vi "Gel Tugging Force Mode_Data Logger v16.20 EPI.vi"() -> ()   [LabVIEW 2015]
uses:
  <vilib>/Utility/error.llb/DialogType.ctl
  <vilib>/DAQmx/read.llb/DAQmx Read (Analog 2D DBL NChan NSamp).vi
  <vilib>/DAQmx/create/channels.llb/DAQmx Create Channel (AI-Voltage-Basic).vi
  <vilib>/DAQmx/configure/timing.llb/DAQmx Timing (Sample Clock).vi
  <vilib>/DAQmx/configure/trigger.llb/DAQmx Start Trigger (Digital Edge).vi
  <vilib>/DAQmx/miscellaneous.llb/DAQmx Fill In Error Info.vi
  <vilib>/Utility/file.llb/Write Delimited Spreadsheet (DBL).vi
  <resource>/objmgr/daqmx.rc
  <resource>/objmgr/ni.dex.rc
panel:
  in  "Filename: 2":string="R1"
  out "Loop Index":i32
  out "Data Points":u64
  in  "Working Directory":path=path "C:/Users/Selby1/Desktop" caption="Path"
  in  "Filename:":string="S20210722_1mgmL_37C-S2-B1-EDC"
  out "Current Plot (V)":dbl[](graph)
  out "Exposure Plot (V)":dbl[](graph)
  out "Flux Plot (V)":dbl[](graph)
  in  "Start Manual Trigger Button":bool
  in  "Trigger Type?":bool=TRUE
  in  "Notes:":string="0.5-µm carboxylate-coated Fluorosphere red beads\n4.5-µm M450 Dynabeads tosylactivated magnetic beads \n0.75 mg/mL type I collagen gel @ 37°C, pH ~7.4. Prepared on 2021-08-17\nNOT Covered with 2.6mM EDAC + 0.1M MES (pH~ 6.0) solution for 30 minutes\n18-mm diameter Sylgard 184 1:10 mixture. Poured 6.2 g onto \"100-mm\" petri dish to create ~750 µm thick molds.\nCoated the gel with 10 µL red bead/mL MilliQ water left for 10-30 seconds. \nWashed the gel before adding the red beads with clean milliQ water\n250 µL of collagen gel mix (~800 µm). Consider using 235 µL next time."
  out "Total Ramp \nTime (ms)":i16
  out "# Ramp\nSteps":i16
  out "Red Fluoroescent Microspheres\nDiameter (Micron)":dbl=0.5 format="%#.1g"
  out "Tip Initial XY Separation\n (micron) Separation\n Distance (micron)":dbl=15.0
  out "Image Scale \n(micron/pixel)":dbl=0.21604
  out "Gel Thickness\n(Micron)":dbl=662.0
  in  "Fluoro Beads \nZ-Level\n(Micron)":dbl
  in  "Magnetic \nBead Z-Level\n(Micron)":dbl
  out "Tip Z-level Above Gel Surface (micron)":dbl=11.0
  out "Digital Trigger":bool
  out "Flux On\n Setpoint (Gs)":dbl=2.4945191 format="%.3g"
  out "Column 4":string="Flux Sensor (V)"
  out "Column 3":string="Flux Sensor (V)"
  out "Column 1":string="Flux Sensor (V)"
  out "Column 2":string="Flux Sensor (V)"
  out "Temperature\n(ºC)":dbl=25.7
  out "Ready?":bool
  in  "?":bool
  out "Relative \nHumidity (%)":dbl=42.0
  out "Magnetic Flux Sensor\n Sensitivity (V/Gs)":dbl=2.4945191 format="%#_8g"
  out "Magnetic Bead\nDiameter (Micron)":dbl=4.5 format="%#.1g"
  out "Needle\n Inclination \nAngle (º)":dbl=25.0
  out "Cycles":i16
  out "Downloading\nData":bool
  out "Magnetic Flux Sensor\n Zero, Crude Mean (V)":dbl=2.4945191 format="%.6g"
  # "For Gel Tugging Experiments v16.20-EPI Part"
  # "Verify Data Further with  \"Gel Tugging Force Mode_Data Reduction v16.00.vi\" or \"ReadSensorData.m\" in MATLAB"
  # "Step 1: Enter:"
  # "-EPI-"
  # ".dat"
  # "&"
  # "_Notes.txt"
  # "Manual"
  # "Automatic"
  # "Step 2: Click TRGR or Run Macro in Nikon Elements"
  # "datapoints downloaded"
  # "out of"
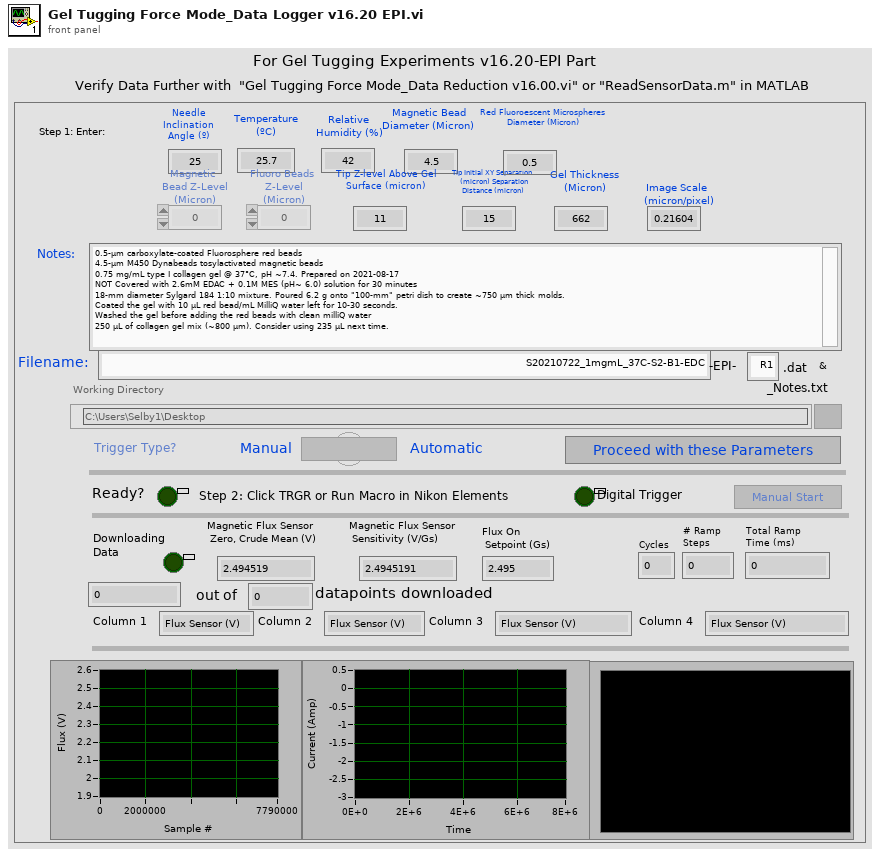
[diagram p1: front panel]
types:
  T1 = enum8{"Enabled", "Disabled", "Disabled and Grayed Out"}
  T2 = typedef "DialogType.ctl" = u16
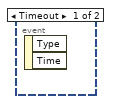
[diagram p2: hidden frame]
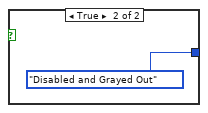
[diagram p3: hidden frame]
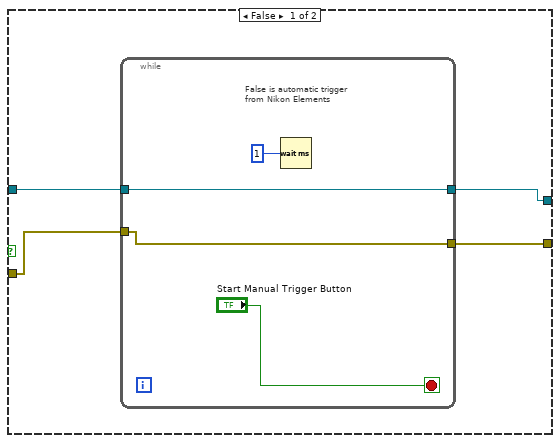
[diagram p4: hidden frame]
diagram:
  # "Modified from v15.00 by #Waddah #Moghram on 12/18/2018 and thereafter.\n1. Added a note section that will be in a file with the same note, but add \"notes\" to it. \n2. Tip -> Magnetic Bead. Magnetic Bead -> Fluorobeads. Fluoro beads -> Tip z-level. Headers were corrected 12/20/2018\n \nModified from v11.00 by #Waddah #Moghram on 5/4/2018 and thereafter:\n1. Updated the header to include gel-related information such as z-levels for the tip, bead, and thickness; gel thickness.\n2. Changed output file extension to *.dat\n3. Added a few other headers. Updated Ramp Step Information 11/28/2018\n\nModified from v10.00 by #Waddah #Moghram on 4/26/2018:\n1. This program will get the digital trigger from Nikon Elements. Then it will forward it to the control sequence VI on the slave DAQ for real-time sequence. This is a roundabout way to deal with the issue of ground loop problems.\n\nModified from v8.00 and later by #Waddah #Moghram on 4/4/2018 \n2. Just add an extra Row...with Null Flux Corrective just for the record. Did not mess with anything previously\n2. \"Flux Observed Zero\" renamed to \"Null Flux Observed\"\n3. \"AO Signal\" is replaced back to \"Camera Exposure (V)\"\n4. Added Labels \"Rows\" to the Header to keep track\n5. Updated Samples read per loop from 400 to 40000 4/1/2018\n6. Added Headers for Gel properties\n\nModified from v7.40 by #Waddah #Moghram on 1/4/2018\n1. Remove Step 0: Recording temperature with thermocouple. Thermocouple reading is not reliable, whether is the one built into labVIEW or the handheld one. Enter the value read by the Digital Thermometer along with relative humidity readings.\n2. Added an extra row to store both sets of PIDs for ON/OFF. \n3. Modified Tabbing Order on 3/4/2018\n4. Added Columns Display at front panel 3/18/2018\n\nModified from v7.30 by #Waddah #Moghram on 12/23/2017\n1. Added event close loop to make the Data Logger Running False if user closes it abruptly. \nNote: Aborting event is not included. Avoid aborting if possible.\n2. corrected total number of data points to allow for more than 2 seconds 1/4/2018 by #WIM\n\nModified from v7.00 by #Waddah #Moghram on 12/21/2017\n1. Reduce Thermocouple time to 1 \n2. Added another Text to record room temperature manual. But be consistent.\n\nModified from v6.00 by #Waddah #Moghram on 12/18/2017\n1. Added Relative Humidity Entry instead of \"Dummy Variable Entry in the Header.\" This value is to be entered from the reading of Relative Humidity\\\n2. Added Thermocouple measurement VI into this one. Average and storage into Data Logger for future purposes. \n\nModified from v5.22 by #Waddah #Moghram on 12/05/2017\n1. Added Entry for Magnetic Sensor Sensitivity\n2. Added Precisions for Header Values\n\nModified from v.4.00 by #Waddah #Moghram on 8/9/2017\n\nModified from v.3.80 by #Waddah #Moghram on 8/7/2017\n*Current Dialog boxes. Use Stacked sequences. Cleaned up v.3.80\n*Included Post  & Pre-wave Periods in Data Collection\n\nModified by #Waddah #Moghram on 8/7/2017\n*Include PID Parameters in the file\n*Modified headers of columns to be able to be extracted from MATLAB\n*Network stream loop is cleaned up \n*Removed Data Logging Time. Whatever it it takes to download the entire stream.\n*works with local single process FIFO\n\nDigital Input (Trigger)\n1. Dev3/PFI0 is connected internally in the DAQ-1/Master Connecter block. It is also wired up to DAQ-2/Slave Connector Block\n\nModifications from previous edition:\n1. Removed AI1 & AI2 to see if instability is due to a ground loop.\n\nNote: Sampling rate for Data Logger is 10,000 Samples/Second"
  n1 = flat-sequence {
    tunnel: [w20] -> w2
    tunnel: [w32] -> w12
    tunnel: [w33] -> w11
    tunnel: w2 -> [w29]
    tunnel: [w29] -> w1
    tunnel: w12 -> [w46]
    tunnel: w11 -> [w45]
    tunnel: [w47] -> w7
    tunnel: [w48] -> w3
    tunnel: w1 -> [w44]
    tunnel: [w228] -> w8
    tunnel: w7 -> [w161]
    tunnel: [w161] -> w6
    tunnel: [w291] -> w5
    tunnel: [w167] -> w4
    tunnel: w3 -> [w291]
    tunnel: w8 -> [w301]
    tunnel: w6 -> [w307]
    tunnel: [w296] -> w10
    tunnel: w5 -> [w306]
    tunnel: [w300] -> w9
    tunnel: w4 -> [w315]
    tunnel: w10 -> [w382]
    tunnel: w9 -> [w381]
    frame #0 {
      (unwired) "1. OPEN the PID Control VI & Follow Instructions **if you have not done so already**.\n2. Click OK to begin temperature measurement & ENTER other variables afterwards.\n3. RUN the macro (if a macro is used). Otherwise, CLICK  \"TRGR\" button in Nikon Elements to initiate Fast Timelapse Image Capture, Data Acquisition, and PID-Controlled Sequence."
      # "Clear Graphs"
      # "Reset the Data Download"
      n2 = shared-variable "NI-GenericDesktopPC-3A84958E\\Kopco PS Project Target Variables Library.lvlib\\DataFolderName"() -> (w14:string)  [unwired: 1 in, 1 out]
      n3 = shared-variable "NI-GenericDesktopPC-3A84958E\\Kopco PS Project Target Variables Library.lvlib\\DataFileName"() -> (w15:string)  [unwired: 1 in, 1 out]
      n4 = shared-variable "NI-GenericDesktopPC-3A84958E\\Kopco PS Project Target Variables Library.lvlib\\Notes"() -> (w19:string)  [unwired: 1 in, 1 out]
      n5 = String To Path(string=w14) -> (path=w13:path)
      n6 = property on="Exposure Plot (V)" class="WFGraph (strict)"("Value"=dbl[] [] ("Current Plot (V)")) -> ()  [unwired: 2 in, 2 out]
      n7 = property on="Current Plot (V)" class="WFGraph (strict)"("Value"=dbl[] [] ("Flux Plot (V)")) -> ()  [unwired: 2 in, 2 out]
      n8 = property on="Flux Plot (V)" class="WFGraph (strict)"("Value"=dbl[] [] ("Exposure Plot (V)")) -> ()  [unwired: 2 in, 2 out]
      n9 = property on="Notes:" class="Str"("Text.Text"=w19) -> ()  [unwired: 2 in, 2 out]
      n10 = property on="Filename:" class="Str"("Text.Text"=w15) -> ()  [unwired: 2 in, 2 out]
      n11 = property on="Working Directory" class="Path"("Value"=w13) -> ()  [unwired: 2 in, 2 out]
    }
    frame #1 {
      # "Gives a pause to adjust the values before confirmation"
      # "Bound to \"Experiment Settings Entered\"\nglobal shared variable."
      n12 = while {
        tunnel: ["?"] -> w21
        tunnel: ["Trigger Type?"] -> w20
        stop <- "?" stop-if-true
        w23 = FALSE ("Data Download")
        n13 = shared-variable "NI-GenericDesktopPC-3A84958E\\Kopco PS Project Target Variables Library.lvlib\\Data Download"(w23) -> ()  [unwired: 1 in, 1 out]
        n14 = shared-variable "NI-GenericDesktopPC-3A84958E\\Kopco PS Project Target Variables Library.lvlib\\Data Logger Running"(TRUE ("Data Logger Running")) -> ()  [unwired: 1 in, 1 out]
        n15 = case shown="False" "Trigger Type?" {
          tunnel: [T1."Enabled" ("Disabled") T1."Disabled and Grayed Out" ("Disabled")] -> w26
          frame False {
          }
          frame True {
          }
        }
        n16 = shared-variable "NI-GenericDesktopPC-3A84958E\\Kopco PS Project Target Variables Library.lvlib\\Temperature Measured"(w23) -> ()  [unwired: 1 in, 1 out]
        n17 = shared-variable "NI-GenericDesktopPC-3A84958E\\Kopco PS Project Target Variables Library.lvlib\\Experiment Settings Entered"(w23) -> ()  [unwired: 1 in, 1 out]
        n18 = shared-variable "NI-GenericDesktopPC-3A84958E\\Kopco PS Project Target Variables Library.lvlib\\Digital Trigger"(w23) -> ()  [unwired: 1 in, 1 out]
        n19 = property on="Start Manual Trigger Button" class="Bool"("Disabled"=w26) -> ()  [unwired: 2 in, 2 out]
      }
      n20 = shared-variable "NI-GenericDesktopPC-3A84958E\\Kopco PS Project Target Variables Library.lvlib\\Experiment Settings Entered"(w21) -> ()  [unwired: 1 in, 1 out]
    }
    frame #2 {
      w30 = 30000.0  # AI Frequency
      w34 = 10106 items=["Default"=-1, "RSE"=10083, "NRSE"=10078, "Differential"=10106, "Pseudodifferential"=12529] ("input terminal configuration")
      w35 = 10123 items=["Finite Samples"=10178, "Continuous Samples"=10123] ("sample mode")
      # "Configuring Analog Inputs (AIs)\n3. Dev2/AI5 is connected to \"RAW\" Magnetic Flux Sensor\n4. Dev2/AI6 is connected to \"Current Senssor (1A/V)\"\n5. Dev2/AI7 is connected to Camera Exposure Signal (\"Out 4\" on sCMOS Camera)"
      # "As of 8/3/2017. This is \njust to initiate digital trigger.\nNo data is collected via master DAQ"
      n21 = call-poly <vilib>:"DAQmx Create Virtual Channel.vi"("maximum value"=10.0, "minimum value"=-10.0, "input terminal configuration"=w34, "physical channels"="Dev3/ai3") -> ("task out"=w37:refnum<k21>, "error out"=w36:errorcluster)  [unwired: 10 in]
      n22 = call-poly <vilib>:"DAQmx Timing.vi"("task/channels in"=w37, "sample mode"=w35, "rate"=w30, "source"=tag "OnboardClock" ("Sample Clock Source"), "error in"=w36) -> ("task out"=w38:refnum<k21>, "error out"=w39:errorcluster)  [unwired: 9 in]
      n23 = call <vilib>:"DAQmx Configure Input Buffer.vi"("task/channels in"=w38, "buffer size (in samples per channel)"=200000, "error in"=w39) -> ("task out"=w32:refnum<k21>, "error out"=w33:errorcluster)  [unwired: 11 in]
    }
    frame #3 {
      n24 = case shown="True" w44 {
        tunnel: [w52 w70] -> w49
        tunnel: w45 -> [w53 w62]
        tunnel: [w55 w61] -> w50
        tunnel: w46 -> [w54 w60]
        frame False {
          n25 = while {
            tunnel: [w58] -> w55
            tunnel: w54 -> [w58]
            tunnel: w53 -> [w57]
            tunnel: [w57] -> w52
            stop <- "Start Manual Trigger Button" stop-if-true
            # "False is automatic trigger \nfrom Nikon Elements"
            n26 = Wait (ms)(milliseconds to wait=u32 1) -> ()  [unwired: 1 out]
          }
        }
        frame True {
          w63 = 10280 items=["Rising"=10280, "Falling"=10171] ("edge")
          # "True is automatic trigger \nfrom Nikon Elements"
          # "Waiting for Digital Trigger (\"TRGR\") from Nikon Element\nOr Macro that has a digital trigger"
          n27 = call-poly <vilib>:"DAQmx Trigger.vi"("task/channels in"=w60, "source"=tag "/Dev3/PFI0", "edge"=w63, "error in"=w62) -> ("task out"=w65:refnum<k21>, "error out"=w67:errorcluster)  [unwired: 10 in]
          n28 = property class="DAQmx Trigger"(reference=w65, error in=w67, "Start.DigEdge.DigFltr.MinPulseWidth"=1e-06) -> (reference out=w66:refnum<k21>, error out=w68:errorcluster)
          n29 = call <vilib>:"DAQmx Start Task.vi"("task/channels in"=w66, "error in"=w68) -> ("task out"=w61:refnum<k21>, "error out"=w70:errorcluster)  [unwired: 12 in]
        }
      }
      n30 = while "Just a one-item loop for to start the digital trigger" {
        tunnel: w49 -> [w77]
        tunnel: w50 -> [w76]
        tunnel: [w75] -> w48
        tunnel: [w74] -> w47
        tunnel: [w71] -> w51
        i -> [w73]
        stop <- w71 stop-if-true
        w79 = -1.0  # timeout
        # "Added on 4/24/2018. Digital Trigger to be transferred to \nRT control sequence VI"
        n31 = Equal?(x=1, y=w73) -> (x = y?=w71:bool)
        n32 = call-poly <vilib>:"DAQmx Read.vi"("task/channels in"=w76, "number of samples per channel"=1, "timeout"=w79, "error in"=w77) -> ("task out"=w75:refnum<k21>, "error out"=w74:errorcluster)  [unwired: 9 in, 1 out]
        n33 = Unbundle By Name(w74) -> ()  [unwired: 1 out]
      }
      n34 = shared-variable "NI-GenericDesktopPC-3A84958E\\Kopco PS Project Target Variables Library.lvlib\\Digital Trigger"(w51) -> ()  [unwired: 1 in, 1 out]
    }
    frame #4 {
      w117 = 0.0  # number
      w133 = "\t"
      w135 = "\t"
      w158 = "\t"
      w157 = "\t"
      w172 = "\t"
      w171 = "\t"
      (unwired) "AO Signal (V)" ("string")
      w192 = "\t"
      w190 = "\t"
      w218 = "\t"
      w216 = "\t"
      w277 = "\t"
      w275 = "\t"
      w243 = "\t"
      w241 = "\t"
      w178 = "Current AO (V)" ("string")
      w257 = "\t"
      w260 = "\t"
      w169 = "Camera Exposure TTL (V)" ("string")
      w254 = "\t"
      w177 = "Current Sensor (V or A)" ("string")
      w253 = "Flux Sensor (V)" ("string")
      # "Added on 3/17/2018\nfor mini DeGauss & \ntuning experiments. \nModify controller Program accordingly.\n4/4/2018. Back to Camera Exposure"
      # "Added on 3/17/2018\nfor mini DeGauss & \ntuning experiments. \nModify controller Program accordingly.\n4/4/2018. Back to Camera Exposure"
      # "Step Duration is changed to \nSampling Rate, 1/5/2018 by WIM"
      # "Sampling Rate (samples/sec)"
      # "Removed (%) on 12/20/2017 @ 6:58 PM.\nIt should not be % since it is alreayd in decimal. Otherwise, it is %"
      # "Changed from (mV/Gs) to (V/Gs) on 7/18/2017"
      # "Modified on 7/19/2017 to Including Sampling Frequency \ninstead of Sampling Rate to minimize round off Error"
      # "3rd Line Header"
      # "Magentic Sensor Sensitivity"
      n35 = shared-variable "NI-GenericDesktopPC-3A84958E\\Kopco PS Project Target Variables Library.lvlib\\Flux Setpoint ON Gs Relative"() -> (w164:dbl)  [unwired: 1 in, 1 out]
      "Flux On\n Setpoint (Gs)" <- w164
      n36 = shared-variable "NI-GenericDesktopPC-3A84958E\\Kopco PS Project Target Variables Library.lvlib\\NeedleInclinationAngle"() -> (w96:dbl)  [unwired: 1 in, 1 out]
      "Needle\n Inclination \nAngle (º)" <- w96
      n37 = shared-variable "NI-GenericDesktopPC-3A84958E\\Kopco PS Project Target Variables Library.lvlib\\MagneticBeadDiameterMicron"() -> (w95:dbl)  [unwired: 1 in, 1 out]
      "Magnetic Bead\nDiameter (Micron)" <- w95
      n38 = shared-variable "NI-GenericDesktopPC-3A84958E\\Kopco PS Project Target Variables Library.lvlib\\Temperature"() -> (w97:dbl)  [unwired: 1 in, 1 out]
      "Temperature\n(ºC)" <- w97
      n39 = shared-variable "NI-GenericDesktopPC-3A84958E\\Kopco PS Project Target Variables Library.lvlib\\Null Flux Pre Period"() -> (w288:dbl)  [unwired: 1 in, 1 out]
      n40 = shared-variable "NI-GenericDesktopPC-3A84958E\\Kopco PS Project Target Variables Library.lvlib\\RelativeHumidity"() -> (w94:dbl)  [unwired: 1 in, 1 out]
      "Relative \nHumidity (%)" <- w94
      n41 = shared-variable "NI-GenericDesktopPC-3A84958E\\Kopco PS Project Target Variables Library.lvlib\\Zero Flux Observed GS"() -> (w287:dbl)  [unwired: 1 in, 1 out]
      n42 = shared-variable "NI-GenericDesktopPC-3A84958E\\Kopco PS Project Target Variables Library.lvlib\\Null Flux Post Period"() -> (w289:dbl)  [unwired: 1 in, 1 out]
      n43 = shared-variable "NI-GenericDesktopPC-3A84958E\\Kopco PS Project Target Variables Library.lvlib\\PID Parameters ON"() -> (w230:dbl[])  [unwired: 1 in, 1 out]
      n44 = shared-variable "NI-GenericDesktopPC-3A84958E\\Kopco PS Project Target Variables Library.lvlib\\Sensor Sensitivity Core"() -> (w213:dbl)  [unwired: 1 in, 1 out]
      "Magnetic Flux Sensor\n Sensitivity (V/Gs)" <- w213
      n45 = shared-variable "NI-GenericDesktopPC-3A84958E\\Kopco PS Project Target Variables Library.lvlib\\Zero Flux Calibrated Core"() -> (w261:dbl)  [unwired: 1 in, 1 out]
      "Magnetic Flux Sensor\n Zero, Crude Mean (V)" <- w261
      n46 = Index Array(array=w230, index=3) -> (element=w290:dbl)
      n47 = Index Array(array=w230, index=4) -> (element=w167:dbl)
      n48 = Index Array(array=w230, index=2) -> (element=w234:dbl)
      n49 = Number To Fractional String "Flux ON Relative Setpoint (Gs)"(number=w164) -> (F-format string=w282:string)  [unwired: 3 in]
      n50 = Number To Fractional String "Flux Observed Zero (Gs)"(number=w287) -> (F-format string=w281:string)  [unwired: 3 in]
      n51 = Index Array(array=w230, index=1) -> (element=w237:dbl)
      n52 = Index Array(array=w230, index=0) -> (element=w239:dbl)
      n53 = Number To Fractional String "Pre- Zero Interval (s)"(number=w288) -> (F-format string=w280:string)  [unwired: 3 in]
      n54 = Number To Fractional String "Post- Zero Interval (s)"(number=w289) -> (F-format string=w276:string)  [unwired: 3 in]
      n55 = Divide(x=w94, y=100.0) -> (x/y=w207:dbl)
      n56 = shared-variable "NI-GenericDesktopPC-3A84958E\\Kopco PS Project Target Variables Library.lvlib\\Cycles"() -> (w273:i16)  [unwired: 1 in, 1 out]
      n57 = shared-variable "NI-GenericDesktopPC-3A84958E\\Kopco PS Project Target Variables Library.lvlib\\PID Parameters OFF"() -> (w176:dbl[])  [unwired: 1 in, 1 out]
      n58 = Number To Fractional String "Proportional Gain (K_c)"(number=w239) -> (F-format string=w249:string)  [unwired: 3 in]
      n59 = Number To Exponential String "Integral Time (T_i, min)"(number=w237) -> (E-format string=w248:string)  [unwired: 3 in]
      n60 = shared-variable "NI-GenericDesktopPC-3A84958E\\Kopco PS Project Target Variables Library.lvlib\\Needle Used"() -> (w179:i8)  [unwired: 1 in, 1 out]
      n61 = Number To Fractional String "Magnetic Sensor Mean, Crude"(number=w261, precision (6)=i16 6) -> (F-format string=w264:string)  [unwired: 2 in]
      n62 = Number To Exponential String "Derivative Time (T_d, min)"(number=w234) -> (E-format string=w247:string)  [unwired: 3 in]
      n63 = Number To Fractional String "Samples Pushed to PID at a time"(number=w290, precision (6)=i16 0) -> (F-format string=w242:string)  [unwired: 2 in]
      n64 = Number To Fractional String "Number of Cycles"(number=w273, precision (6)=i16 0 ("width (-)")) -> (F-format string=w262:string)  [unwired: 2 in]
      n65 = Number To Fractional String "Sampling Rate (Samples/Sec)"(number=w167, precision (6)=i16 0) -> (F-format string=w256:string)  [unwired: 2 in]
      n66 = Number To Fractional String "Mean Temperature (ºC)"(number=w97, precision (6)=i16 1) -> (F-format string=w223:string)  [unwired: 2 in]
      n67 = Number To Fractional String "Inclination Angle (º)"(number=w96, precision (6)=i16 0) -> (F-format string=w222:string)  [unwired: 2 in]
      n68 = Number To Fractional String "Relative Humidity (%)"(number=w207, precision (6)=i16 2 ("width (-)")) -> (F-format string=w217:string)  [unwired: 2 in]
      n69 = Number To Fractional String "Magnetic Bead Diameter (Micron)"(number=w95, precision (6)=i16 1) -> (F-format string=w221:string)  [unwired: 2 in]
      n70 = Number To Fractional String "Magnetic Sensor Sensitivity"(number=w213, precision (6)=i16 7) -> (F-format string=w263:string)  [unwired: 2 in]
      n71 = Index Array(array=w176, index=2) -> (element=w183:dbl)
      n72 = Index Array(array=w176, index=1) -> (element=w186:dbl)
      n73 = Index Array(array=w176, index=0) -> (element=w188:dbl)
      n74 = Concatenate Strings "1st Row"("Magnetic Sensor Zero (V)" ("string"), w260, "Magnetic Sensor Sensitivity (V/Gs)" ("string"), w260, "Number of Cycles" ("string"), w260, "Sampling Rate (Samples/Sec)" ("string"), "\r") -> (w265:string)
      n75 = Number To Fractional String "OFF Proportional Gain (K_c)"(number=w188) -> (F-format string=w198:string)  [unwired: 3 in]
      n76 = Number To Exponential String "Integral Time (T_i, min)"(number=w186) -> (E-format string=w197:string)  [unwired: 3 in]
      n77 = Number To Exponential String "Derivative Time (T_d, min)"(number=w183) -> (E-format string=w196:string)  [unwired: 3 in]
      n78 = Number To Fractional String "Needle Used"(number=w179, precision (6)=i16 0) -> (F-format string=w191:string)  [unwired: 2 in]
      n79 = shared-variable "NI-GenericDesktopPC-3A84958E\\Kopco PS Project Target Variables Library.lvlib\\TipZaboveGelMicron"() -> (w92:dbl)  [unwired: 1 in, 1 out]
      "Tip Z-level Above Gel Surface (micron)" <- w92
      n80 = Concatenate Strings "2nd Row"(w265, w264, w257, w263, w257, w262, w257, w256, "\r") -> (w233:string)
      n81 = Concatenate Strings "3rd Row"(w233, "ON Proportional Gain (K_c)" ("string"), w241, " Integral Time (T_i, min)" ("string"), w241, "Derivative Time (T_d, min)" ("string"), w241, "Samples pushed to PID" ("string"), "\r") -> (w250:string)
      n82 = Concatenate Strings "4th Row"(w250, w249, w243, w248, w243, w247, w243, w242, "\r") -> (w181:string)
      n83 = Concatenate Strings "5th Row"(w181, "OFF Proportional Gain (K_c)" ("string"), w190, "Integral Time (T_i, min)" ("string"), w190, "Derivative Time (T_d, min)" ("string"), w190, "Needle Used" ("string"), "\r") -> (w199:string)
      n84 = shared-variable "NI-GenericDesktopPC-3A84958E\\Kopco PS Project Target Variables Library.lvlib\\Zero Flux Observed Gs Corrected"() -> (w165:dbl)  [unwired: 1 in, 1 out]
      n85 = shared-variable "NI-GenericDesktopPC-3A84958E\\Kopco PS Project Target Variables Library.lvlib\\TipBeadXYSeparationMicron"() -> (w91:dbl)  [unwired: 1 in, 1 out]
      "Tip Initial XY Separation\n (micron) Separation\n Distance (micron)" <- w91
      n86 = Concatenate Strings "6th Row"(w199, w198, w192, w197, w192, w196, w192, w191, "\r") -> (w180:string)
      n87 = Concatenate Strings "7th Row"(w180, "Flux ON Relative Setpoint (Gs)" ("string"), w275, "Null Flux - Observed (Gs)" ("string"), w275, "Pre-Zero Interval (s)" ("string"), w275, "Post-Zero Interval (s)" ("string"), "\r") -> (w283:string)
      n88 = Concatenate Strings "8th Row"(w283, w282, w277, w281, w277, w280, w277, w276, "\r") -> (w214:string)
      n89 = Concatenate Strings "9th Row"(w214, "Temperature (ºC)" ("string"), w216, "Needle Inclination Angle (º)" ("string"), w216, "Magnetic Beads Diameter (Micron)" ("string"), w216, "Relative Humidity" ("string"), "\r") -> (w224:string)
      n90 = Concatenate Strings "10th Row"(w224, w223, w218, w222, w218, w221, w218, w217, "\r") -> (w168:string)
      n91 = Concatenate Strings "11th Row"(w168, "Null Flux Corrected (Gs)" ("string"), w171, "=====================" ("string"), w171, "=====================" ("string"), w171, "Tip Z-level Above Gel Surface (Micron)" ("string"), "\r") -> (w166:string)
      n92 = Number To Fractional String "Mag bead\n Z-Level\n(Micron)"(number="Magnetic \nBead Z-Level\n(Micron)", precision (6)=i16 2) -> (F-format string=w139:string)  [unwired: 2 in]
      n93 = Number To Fractional String "Tip Z-Above Gel Surface\n(Micron)"(number=w92, precision (6)=i16 2) -> (F-format string=w137:string)  [unwired: 2 in]
      n94 = shared-variable "NI-GenericDesktopPC-3A84958E\\Kopco PS Project Target Variables Library.lvlib\\FrameScaleMicronPerPixel"() -> (w89:dbl)  [unwired: 1 in, 1 out]
      "Image Scale \n(micron/pixel)" <- w89
      n95 = Number To Fractional String "Fluoro Z-Level\n(Micron)"(number="Fluoro Beads \nZ-Level\n(Micron)", precision (6)=i16 2) -> (F-format string=w138:string)  [unwired: 2 in]
      n96 = Number To Fractional String "Null Flux Corrected (GS)"(number=w165) -> (F-format string=w175:string)  [unwired: 3 in]
      n97 = shared-variable "NI-GenericDesktopPC-3A84958E\\Kopco PS Project Target Variables Library.lvlib\\Ramp Total Interval (ms)"() -> (w116:dbl)  [unwired: 1 in, 1 out]
      "Total Ramp \nTime (ms)" <- w116
      n98 = shared-variable "NI-GenericDesktopPC-3A84958E\\Kopco PS Project Target Variables Library.lvlib\\FluorescentMicrospheresDiameterMicron"() -> (w93:dbl)  [unwired: 1 in, 1 out]
      "Red Fluoroescent Microspheres\nDiameter (Micron)" <- w93
      n99 = shared-variable "NI-GenericDesktopPC-3A84958E\\Kopco PS Project Target Variables Library.lvlib\\Ramp Steps"() -> (w115:i16)  [unwired: 1 in, 1 out]
      "# Ramp\nSteps" <- w115
      n100 = Concatenate Strings "12th Row"(w166, w175, w172, w139, w172, w138, w172, w137, "\r") -> (w154:string)
      n101 = Concatenate Strings "13th Row"(w154, "Gel Measured Thickness (Micron)" ("string"), w157, "Initial Separation Distance (Micron)" ("string"), w157, "Frame Scale (micron/pixel)" ("string"), w157, "Fluoro Beads Diameter (Micron)" ("string"), "\r") -> (w155:string)
      n102 = Number To Fractional String "Image Scale\n (micron/pixel)"(number=w89, precision (6)=i16 5) -> (F-format string=w152:string)  [unwired: 2 in]
      n103 = shared-variable "NI-GenericDesktopPC-3A84958E\\Kopco PS Project Target Variables Library.lvlib\\FluorescentMicrospheresDiameterMicron"() -> ()  [unwired: 1 in, 2 out]
      n104 = shared-variable "NI-GenericDesktopPC-3A84958E\\Kopco PS Project Target Variables Library.lvlib\\GelThicknessMicron"() -> (w90:dbl)  [unwired: 1 in, 1 out]
      "Gel Thickness\n(Micron)" <- w90
      n105 = Number To Fractional String "Initial Separation\nDistance (micron)"(number=w91, precision (6)=i16 2) -> (F-format string=w151:string)  [unwired: 2 in]
      n106 = Number To Fractional String(number=w115, precision (6)=i16 0) -> (F-format string=w125:string)  [unwired: 2 in]
      n107 = Number To Fractional String(number=w116, precision (6)=i16 0) -> (F-format string=w124:string)  [unwired: 2 in]
      n108 = Number To Fractional String(number=w117, precision (6)=i16 1) -> (F-format string=w123:string)  [unwired: 2 in]
      n109 = Number To Fractional String(number=w117, precision (6)=i16 1) -> (F-format string=w122:string)  [unwired: 2 in]
      n110 = Number To Fractional String "Gel Measured Thickness (Micron)"(number=w90, precision (6)=i16 2) -> (F-format string=w150:string)  [unwired: 2 in]
      n111 = Number To Fractional String "Fluoro Beads Diameter (Micron)"(number=w93, precision (6)=i16 1) -> (F-format string=w153:string)  [unwired: 2 in]
      n112 = Concatenate Strings("Filename:", "-EPI-" ("string"), "Filename: 2") -> (w86:string)
      n113 = Concatenate Strings "14th Row"(w155, w150, w158, w151, w158, w152, w158, w153, "\r") -> (w128:string)
      n114 = Concatenate Strings "15th Row"(w128, "Ramp Steps" ("string"), w133, "Total Ramp Time (ms)" ("string"), w133, "===============" ("string"), w133, "===============" ("string"), "\r") -> (w127:string)
      n115 = Concatenate Strings "16th Row"(w127, w125, w135, w124, w135, w123, w135, w122, "\r") -> (w126:string)
      n116 = Concatenate Strings(w86, "_Notes") -> (w111:string)
      n117 = Concatenate Strings "note file name"(w111, ".txt" ("string")) -> (w81:string)
      n118 = Concatenate Strings "data file name"(w86, ".dat") -> (w84:string)
      n119 = Get Date/Time String() -> (date string=w107:string, time string=w105:string)  [unwired: 3 in]
      n120 = Concatenate Strings "Notes\nData Header"("Notes for \"", w84, "\" collected on " ("string"), w107, " at " ("string"), w105, ":" ("string"), "\r", "Notes:") -> (w104:string)
      n121 = Build Path(base path="Working Directory", name or relative path=w84) -> (appended path=w85:path)
      n122 = Build Path(base path="Working Directory", name or relative path=w81) -> (appended path=w82:path)
      n123 = Write to Text File(file (use dialog)=w82, text=w104) -> (refnum out=w114:refnum<file>, error out=w113:errorcluster)  [unwired: 2 in, 1 out]
      n124 = Concatenate Strings "17th Row\nData Header"(w126, w178, w254, w253, w254, w177, w254, w169, "\r") -> (w269:string)
      n125 = Close File(refnum=w114, error in=w113) -> ()  [unwired: 2 out]
      n126 = Write to Text File(file (use dialog)=w85, text=w269) -> (refnum out=w270:refnum<file>, error out=w271:errorcluster)  [unwired: 2 in, 1 out]
      n127 = Close File(refnum=w270, error in=w271) -> (path=w228:path)  [unwired: 1 out]
      "Column 2" <- w253
      "Column 1" <- w178
      "Column 3" <- w177
      "Column 4" <- w169
    }
    frame #5 {
      w293 = 4.0  # 4 columns
      w303 = 40000  # Samples Read per loop
      # "100000000 from 36000000 on 3/31/2018"
      # "For 2 minutes"
      # "Note: Each Step is a second"
      # "Sampling Rate (Samples per second)"
      # "I.P. Address of\nRemote Desktop"
      n128 = shared-variable "NI-GenericDesktopPC-3A84958E\\Kopco PS Project Target Variables Library.lvlib\\Period Per Cycle"() -> (w308:dbl)  [unwired: 1 in, 1 out]
      n129 = shared-variable "NI-GenericDesktopPC-3A84958E\\Kopco PS Project Target Variables Library.lvlib\\Null Flux Post Period"() -> (w313:dbl)  [unwired: 1 in, 1 out]
      n130 = shared-variable "NI-GenericDesktopPC-3A84958E\\Kopco PS Project Target Variables Library.lvlib\\Null Flux Pre Period"() -> (w314:dbl)  [unwired: 1 in, 1 out]
      n131 = shared-variable "NI-GenericDesktopPC-3A84958E\\Kopco PS Project Target Variables Library.lvlib\\Cycles"() -> (w309:i16)  [unwired: 1 in, 1 out]
      "Cycles" <- w309
      n132 = Multiply "Total Cycles (s)"(x=w309, y=w308) -> (x*y=w311:dbl)
      n133 = Add "Pre&Post (s)"(x=w314, y=w313) -> (x+y=w310:dbl)
      n134 = shared-variable "NI-GenericDesktopPC-3A84958E\\Kopco PS Project Target Variables Library.lvlib\\Samples Total"() -> (w292:u64)  [unwired: 1 in, 1 out]
      "Data Points" <- w292
      n135 = Add "Total Time\n(s)"(x=w311, y=w310) -> (x+y=w312:dbl)
      n136 = Multiply "Samples per column"(x=w312, y=w315) -> ()  [unwired: 1 out]
      n137 = Multiply "Total # of \nSamples"(x=w293, y=w292) -> (x*y=w320:dbl)
      n138 = Divide "Number of Loops"(x=w320, y=w303) -> (x/y=w302:dbl)
      n139 = Create Network Stream Reader Endpoint(7:100000000 ("reader buffer size"), 9:0.0 ("Double"), 10:"//169.254.136.220/FluxWriter" ("writer url"), 11:"FluxReader" ("reader name")) -> (0:w304:errorcluster, 3:w305:refnum<k21>)  [unwired: 3 in]
      n140 = while {
        tunnel: w305 -> [w322]
        tunnel: w304 -> [w366]
        tunnel: [w365] -> w298
        tunnel: [w364] -> w299
        tunnel: w301 -> [w361]
        tunnel: w307 -> [w367]
        tunnel: [w367] -> w297
        tunnel: w302 -> [_]
        tunnel: w306 -> [w351]
        tunnel: [w351] -> w300
        shift-right: [w333] -> w295
        shift-left: _ -> [w346]
        shift-right: [w334] -> w294
        shift-left: _ -> [w343]
        tunnel: w303 -> [w330]
        tunnel: w293 -> [w326]
        tunnel: w292 -> [w325]
        i -> [w354]
        stop <- w323 stop-if-true
        w335 = 90000  # y
        # "Error 314220 is \nsometimes caused, \nbut all the data should\nbe available once the \nstream is flushed on the other side"
        # "Bound to \"Data Download\""
        # "Delete First 0's from Network Stream"
        # "Offset by Samples Taken Per loop to stop at exactly the right amount of samples\nThe last dialog box is invisible for whatever reason. To find it, Search (CTRL+F) \"TRGR\", and then \nclick \"GO TO\" the first choice. Type an arrow key. 8/8/2017"
        n141 = shared-variable-read ("Read Multiple Elements from Stream")(w322, w366, w330) -> (w365:refnum<k21>, w364:errorcluster, w360:dbl[])  [unwired: 1 in, 1 out]
        n142 = Decimate 1D Array "Input is interleaved"(w360) -> (w359:dbl[], w350:dbl[], w358:dbl[], w349:dbl[])
        n143 = Equal?(x=0, y=w354) -> (x = y?=w355:bool)
        n144 = Build Array(w359, w350, w358, w349) -> (w353:dbl[][])
        n145 = property class="Network Stream Endpoint"(reference=w322) -> ("TotalElmntsWritten"=w328:u64)  [unwired: 1 in, 2 out]
        n146 = Transpose 2D Array(2D array=w353) -> (transposed array=w356:dbl[][])
        n147 = case shown="True" w355 {
          tunnel: w356 -> [w375 w377]
          tunnel: [w375 w376] -> w348
          frame False {
          }
          frame True {
            n148 = Delete From Array(array=w377, length=1, index (row)=0) -> (array with subset deleted=w376:dbl[][])  [unwired: 1 in, 1 out]
          }
        }
        n149 = Transpose 2D Array(2D array=w348) -> (transposed array=w340:dbl[][])
        n150 = Quotient & Remainder(x=w328, y=w326) -> (floor(x/y)=w327:dbl)  [unwired: 1 out]
        n151 = call-poly <vilib>:"Write Delimited Spreadsheet.vi"("file path (dialog if empty)"=w361, "format (%.3f)"="%#.6g", "2D data"=w348, "append to file? (F)"=TRUE) -> ()  [unwired: 10 in, 2 out]
        n152 = Delete From Array(array=w340, index (row)=1 ("index")) -> (deleted portion=w347:dbl[])  [unwired: 2 in, 1 out]
        n153 = Decrement(x=w327) -> (x-1=w324:dbl)
        "Loop Index" <- w324
        n154 = Greater Or Equal?(x=w324, y=w325) -> (x >= y?=w323:bool)
        n155 = Delete From Array(array=w340, index (row)=2 ("index")) -> (deleted portion=w344:dbl[])  [unwired: 2 in, 1 out]
        n156 = Delete From Array(array=w340, index (row)=3 ("index")) -> (deleted portion=→"Exposure Plot (V)":dbl[])  [unwired: 2 in, 1 out]
        n157 = Build Array (concatenate)(w346, w347) -> (w339:dbl[])
        n158 = Build Array (concatenate)(w343, w344) -> (w338:dbl[])
        n159 = Not(x=w323) -> (.not. x?=w352:bool)
        n160 = Array Size(array=w338) -> (size(s)=w337:i32)
        n161 = Less?(x=w337, y=w335) -> (x < y?=w336:bool)
        n162 = Multiply(x=2, y=w330) -> (x*y=w332:i32)
        n163 = case shown="True" w336 {
          tunnel: [w369 w370] -> w334
          tunnel: w338 -> [w369 w374]
          tunnel: w339 -> [w368 w373]
          tunnel: [w368 w371] -> w333
          tunnel: w332 -> [_ w372]
          frame False {
          }
          frame True {
            n164 = Delete From Array(array=w374, length=w372) -> (deleted portion=w370:dbl[])  [unwired: 1 in, 1 out]
            n165 = Delete From Array(array=w373, length=w372) -> (deleted portion=w371:dbl[])  [unwired: 1 in, 1 out]
          }
        }
        n166 = shared-variable "NI-GenericDesktopPC-3A84958E\\Kopco PS Project Target Variables Library.lvlib\\Data Download"(w352) -> ()  [unwired: 1 in, 1 out]
      }
      "Flux Plot (V)" <- w295
      "Current Plot (V)" <- w294
      n167 = Destroy Stream Endpoint(8:w299, 11:w298) -> (0:w321:errorcluster)
      n168 = Merge Errors(w297, w321) -> (w296:errorcluster)
    }
    frame #6 {
      w380 = FALSE ("Data Logger Running")
      w386 = T2 3 items=["no dialog", "OK message", "continue or stop message", "OK message + warnings", "continue/stop + warnings"] ("type of dialog (OK msg:1)")
      n169 = call <vilib>:"DAQmx Stop Task.vi"("task/channels in"=w381, "error in"=w382) -> ("task out"=w385:refnum<k21>, "error out"=w384:errorcluster)  [unwired: 12 in]
      n170 = shared-variable "NI-GenericDesktopPC-3A84958E\\Kopco PS Project Target Variables Library.lvlib\\Temperature Measured"(w380) -> ()  [unwired: 1 in, 1 out]
      n171 = shared-variable "NI-GenericDesktopPC-3A84958E\\Kopco PS Project Target Variables Library.lvlib\\Experiment Settings Entered"(w380) -> ()  [unwired: 1 in, 1 out]
      n172 = shared-variable "NI-GenericDesktopPC-3A84958E\\Kopco PS Project Target Variables Library.lvlib\\Data Logger Running"(w380) -> ()  [unwired: 1 in, 1 out]
      n173 = shared-variable "NI-GenericDesktopPC-3A84958E\\Kopco PS Project Target Variables Library.lvlib\\Digital Trigger"(w380) -> ()  [unwired: 1 in, 1 out]
      n174 = call <vilib>:"DAQmx Clear Task.vi"("task in"=w385, "error in"=w384) -> ("error out"=w383:errorcluster)  [unwired: 13 in]
      n175 = call <vilib>:"Simple Error Handler.vi"("type of dialog (OK msg:1)"=w386, "error in (no error)"=w383) -> ()  [unwired: 3 in, 5 out]
    }
    frame #7 {
      (unwired) "OK!"
      (unwired) "1. TURN OFF \"TRGR\" if clicked inside Nikon Elements\n2. VERIFY that the \"Number of Data Points\" matches the number displayed in the \n\"Reduction for Data Logger on Host Computer Triggered by Nikon Elements v16.00 Gel.vi\"  (It should be one sample more than the latest index)."
    }
    frame #8 {
      n176 = Stop() -> ()  [unwired: 1 in]
    }
  }
  n177 = event shown="[1] Panel Close?" {
    selector: _ -> [_ _]
    dyn-events: _ -> [_ _]
    timeout: _ -> [_ _]
    event Timeout {
      n178 = event-data() -> ()  [unwired: 1 in, 2 out]
    }
    event Panel Close? {
      n179 = event-data() -> ()  [unwired: 1 in, 3 out]
      n180 = shared-variable "NI-GenericDesktopPC-3A84958E\\Kopco PS Project Target Variables Library.lvlib\\Data Logger Running"(FALSE ("Data Logger Running")) -> ()  [unwired: 1 in, 1 out]
      n181 = event-data() -> ()  [unwired: 2 in, 1 out]
    }
  }
